vi "Translate Core.vi"(8 "error in (no error)":errorcluster, 10 "Translation":T1, 11 "Layered Shape in":refnum<class "Layered Shape.lvclass">) -> (0 "error out":errorcluster, 3 "Layered Shape out":refnum<class "Layered Shape.lvclass">)   [LabVIEW 2015, in "LV Image Editor Framework.lvlib" / "Layered Shape.lvclass"]
uses:
  Layered Shape.lvclass
  <vilib>/Utility/miscctls.llb/LVPoint32TypeDef.ctl
  Shape/Shape.lvclass
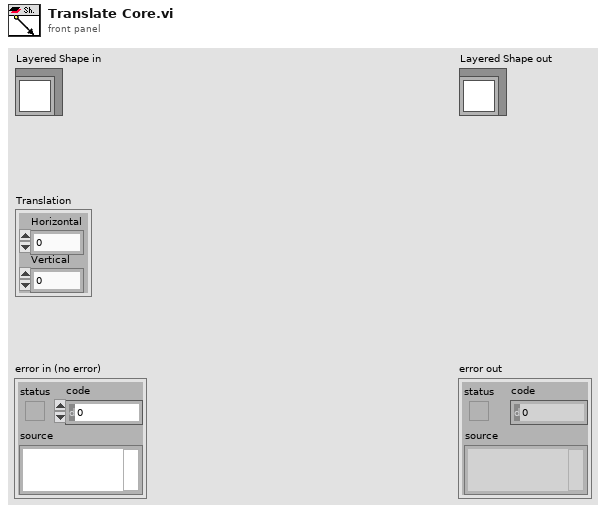
[diagram p1: front panel]
types:
  T1 = typedef "LVPoint32TypeDef.ctl" = cluster{"Horizontal":i32, "Vertical":i32}
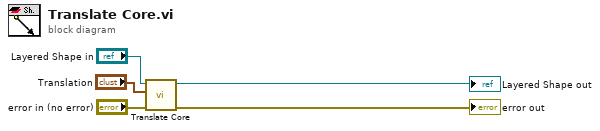
[diagram p0: block diagram]
diagram:
  n1 = call-parent "Translate Core.vi"("error in (no error)"="error in (no error)", "Translation"="Translation", "Shape in"="Layered Shape in") -> ("error out"=→"error out":errorcluster, "Shape out"=→"Layered Shape out":refnum<class "Layered Shape.lvclass">)  [unwired: 7 in]
